vi "Stitch on X axis.vi"(7 "Enum":T1(ring), 8 "error in (no error)":errorcluster, 9 "Right Video":T2, 10 "Initial frame":bool, 11 "Left Video":T2) -> (0 "error out":errorcluster, 3 "Resulting video":T2)   [LabVIEW 2013]
uses:
  <vilib>/vision/Image Controls.llb/IMAQ Image.ctl
  <vilib>/vision/NI_Vision_Development_Module.lvlib
panel:
  # "RE-ENTRANT VI"
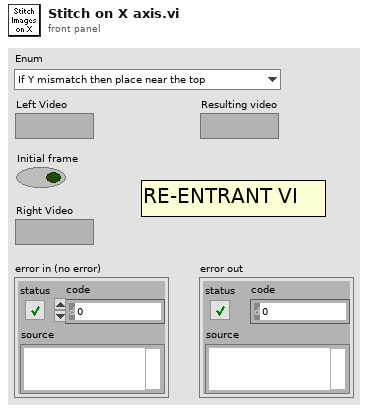
[diagram p1: front panel]
types:
  T1 = enum16{"If Y mismatch then place near the top", "If Y mismatch then place near the bottom"}
  T2 = typedef "IMAQ Image.ctl" = refnum<image>
  T3 = typedef "Image Type" = u32
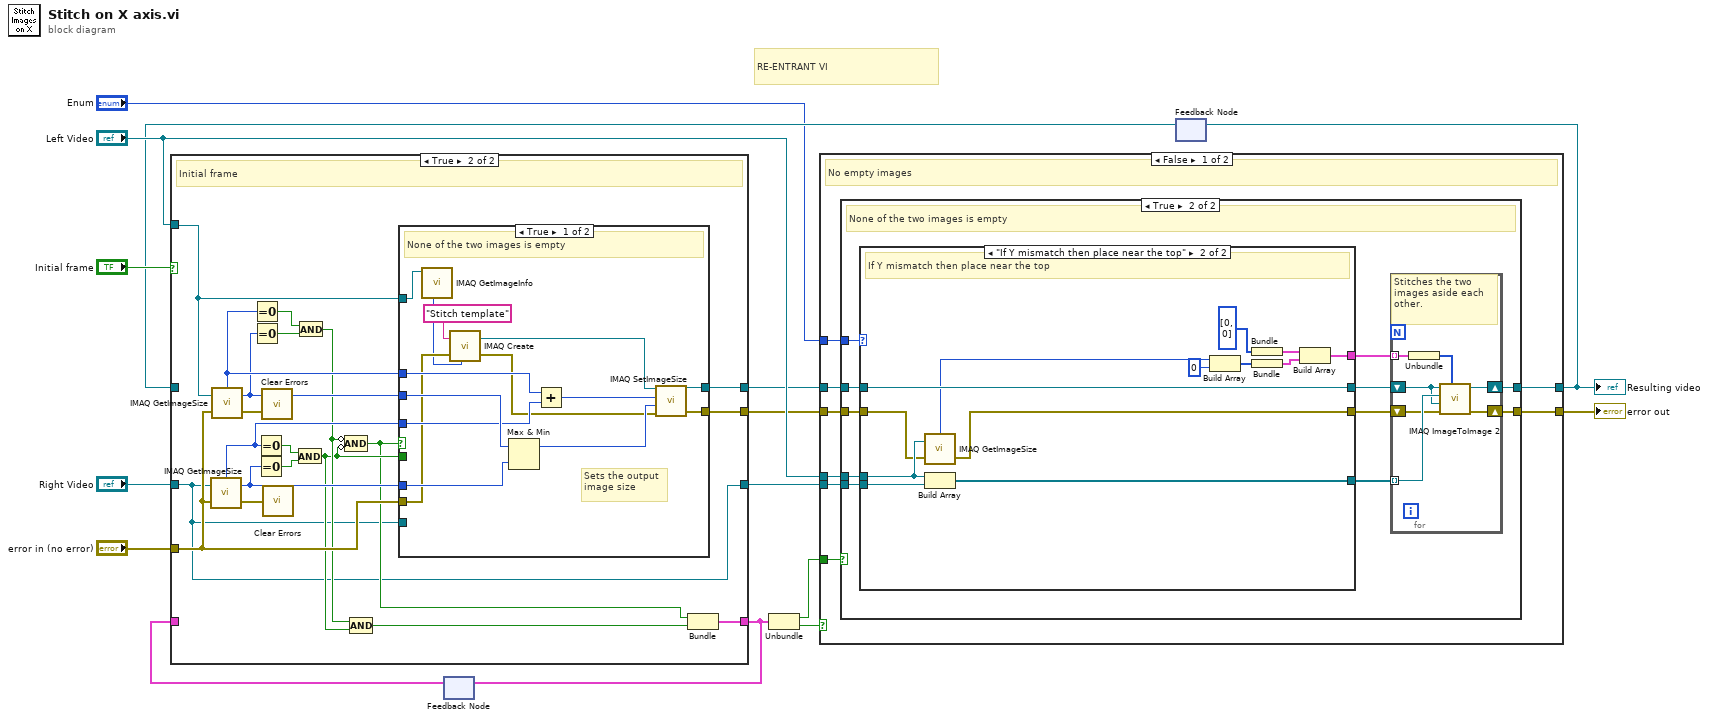
[diagram p0: block diagram]
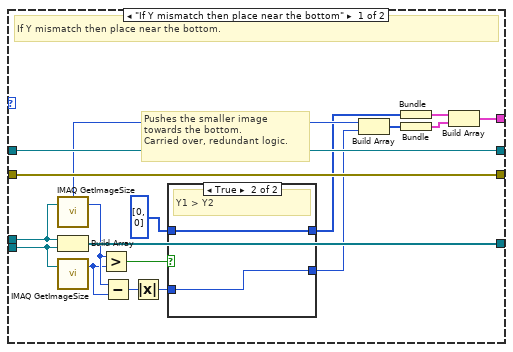
[diagram p3: hidden frame]
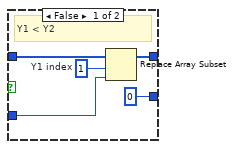
[diagram p4: hidden frame]
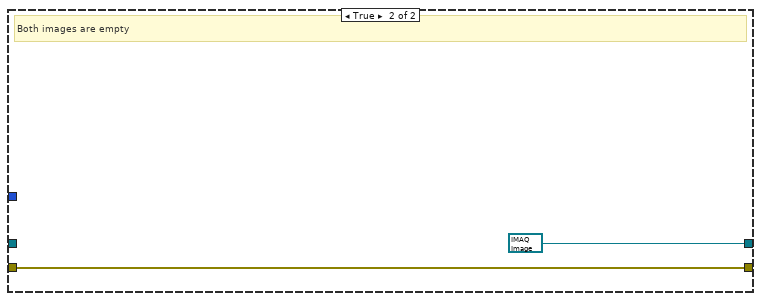
[diagram p5: hidden frame]
diagram:
  # "RE-ENTRANT VI"
  n1 = feedback #1() -> (w8:cluster{bool, bool})  [unwired: 1 in]
  n2 = feedback #2() -> (w7:T2)  [unwired: 1 in]
  n3 = case shown="True" "Initial frame" {
    tunnel: "error in (no error)" -> [w19 w29]
    tunnel: [w19 w38] -> w2
    tunnel: [w18 w39] -> w3
    tunnel: [w17 w20] -> w4
    tunnel: w7 -> [w18 _]
    tunnel: "Right Video" -> [w17 w20]
    tunnel: "Left Video" -> [_ w21]
    tunnel: w8 -> [w16 _]
    tunnel: [w16 w22] -> w9
    frame False {
      # "Default..."
    }
    frame True {
      # "Initial frame"
      n4 = call "IMAQ GetImageSize"("Image"=w20, "error in (no error)"=w29) -> ("Y Resolution"=w31:i32, "X Resolution"=w30:i32, "error out"=w28:errorcluster)  [unwired: 2 in]
      n5 = call "IMAQ GetImageSize"("Image"=w21, "error in (no error)"=w29) -> ("Y Resolution"=w36:i32, "X Resolution"=w37:i32, "error out"=w27:errorcluster)  [unwired: 2 in]
      n6 = Equal To 0?(x=w37) -> (x = 0?=w35:bool)
      n7 = Equal To 0?(x=w36) -> (x = 0?=w34:bool)
      n8 = Equal To 0?(x=w30) -> (x = 0?=w33:bool)
      n9 = Equal To 0?(x=w31) -> (x = 0?=w32:bool)
      n10 = call <vilib>:"Clear Errors.vi"("error in (no error)"=w27) -> ()  [unwired: 6 in, 1 out]
      n11 = call <vilib>:"Clear Errors.vi"("error in (no error)"=w28) -> ()  [unwired: 6 in, 1 out]
      n12 = And(x=w33, y=w32) -> (x .and. y?=w25:bool)
      n13 = And(x=w35, y=w34) -> (x .and. y?=w26:bool)
      n14 = Compound Arithmetic op=AND(invert w26, invert w25) -> (w24:bool)
      n15 = Compound Arithmetic op=AND(w26, w25) -> (w23:bool)
      n16 = case shown="True" w24 {
        tunnel: [w53 w63] -> w39
        tunnel: w29 -> [w43 w62]
        tunnel: [w52 w61] -> w38
        tunnel: w37 -> [w51 w60]
        tunnel: w36 -> [w50 w59]
        tunnel: w31 -> [w49 w58]
        tunnel: w30 -> [w48 w57]
        tunnel: w25 -> [_ w56]
        tunnel: w21 -> [w41 w55]
        tunnel: w20 -> [_ w54]
        frame True {
          # "Sets the output image size"
          # "None of the two images is empty"
          n17 = call "IMAQ GetImageInfo"("Image"=w41) -> ("Image Type"=w40:T3)  [unwired: 3 in, 7 out]
          n18 = call "IMAQ Create"("Image Name"="Stitch template", "Image Type"=w40, "error in (no error)"=w43) -> ("New Image"=w45:T2, "error out"=w44:errorcluster)  [unwired: 1 in, 1 out]
          n19 = Max & Min(x=w50, y=w49) -> (max(x,y)=w46:i32)  [unwired: 1 out]
          n20 = Add(x=w51, y=w48) -> (x+y=w47:i32)
          n21 = call "IMAQ SetImageSize"("error in (no error)"=w44, "Y Resolution"=w46, "X Resolution"=w47, "Image"=w45) -> ("error out"=w52:errorcluster, "Image Out"=w53:T2)  [unwired: 1 out]
        }
        frame False {
          # "One or both images are empty."
          n22 = case shown="True" w56 {
            tunnel: [w65 w66] -> w63
            tunnel: w62 -> [w64 w67]
            tunnel: [w64 w67] -> w61
            tunnel: w60 -> [_ _]
            tunnel: w59 -> [_ _]
            tunnel: w58 -> [_ _]
            tunnel: w57 -> [_ _]
            tunnel: w55 -> [_ w66]
            tunnel: w54 -> [w65 _]
            frame False {
            }
            frame True {
            }
          }
        }
      }
      n23 = Bundle(w24, w23) -> (w22:cluster{bool, bool})  [unwired: 1 in]
    }
  }
  n24 = feedback-in #1(w9) -> ()
  n25 = Unbundle(w9) -> (w10:bool, w11:bool)
  n26 = case shown="False" w11 {
    tunnel: w2 -> [w75 w135]
    tunnel: w3 -> [w74 _]
    tunnel: "Left Video" -> [w73 _]
    tunnel: w4 -> [w72 _]
    tunnel: [w71 w135] -> w5
    tunnel: [w70 T2 refnum ("Selected image")] -> w6
    tunnel: w10 -> [w69 _]
    tunnel: "Enum" -> [w68 _]
    frame False {
      # "No empty images"
      n27 = case shown="True" w69 {
        tunnel: w75 -> [w76 w80]
        tunnel: w74 -> [w77 w82]
        tunnel: w73 -> [_ w85]
        tunnel: w72 -> [_ w84]
        tunnel: [w76 w87] -> w71
        tunnel: [w77 w86] -> w70
        tunnel: w68 -> [_ w78]
        frame False {
          # "One of the images is empty"
        }
        frame True {
          # "None of the two images is empty"
          n28 = case shown="\"If Y mismatch then place near the top\"" w78 {
            tunnel: [w106 w126] -> w88
            tunnel: w85 -> [w105 w125]
            tunnel: w84 -> [w104 w124]
            tunnel: [w103 w123] -> w83
            tunnel: w82 -> [w102 w122]
            tunnel: [w102 w122] -> w81
            tunnel: w80 -> [w101 w121]
            tunnel: [w101 w120] -> w79
            frame "If Y mismatch then place near the bottom" {
              # "Pushes the smaller image towards the bottom.\nCarried over, redundant logic."
              # "If Y mismatch then place near the bottom."
              n29 = call "IMAQ GetImageSize"("Image"=w105) -> ("Y Resolution"=w99:i32, "X Resolution"=w94:i32)  [unwired: 1 in, 3 out]
              n30 = Build Array(w105, w104) -> (w106:T2[])
              n31 = call "IMAQ GetImageSize"("Image"=w104) -> ("Y Resolution"=w98:i32)  [unwired: 1 in, 4 out]
              n32 = Greater?(x=w99, y=w98) -> (0:w100:bool)
              n33 = Subtract(x=w99, y=w98) -> (x-y=w97:i32)
              n34 = Absolute Value(x=w97) -> (abs(x)=w96:i32)
              n35 = case shown="True" w100 {
                tunnel: i32[] [0, 0] -> [w110 w113]
                tunnel: [w109 w113] -> w91
                tunnel: w96 -> [w108 w112]
                tunnel: [0 ("new element/subarray") w112] -> w93
                frame False {
                  w111 = 1  # Y1 index
                  # "Y1 < Y2"
                  n36 = Replace Array Subset(array=w110, new element=w108, index=w111) -> (w109:i32[])
                }
                frame True {
                  # "Y1 > Y2"
                }
              }
              n37 = Build Array(w94, w93) -> (w92:i32[])
              n38 = Bundle(w91) -> (w89:cluster{i32[]})  [unwired: 1 in]
              n39 = Bundle(w92) -> (w90:cluster{i32[]})  [unwired: 1 in]
              n40 = Build Array(w89, w90) -> (w103:cluster{i32[]}[])
            }
            frame "If Y mismatch then place near the top" {
              # "If Y mismatch then place near the top"
              n41 = call "IMAQ GetImageSize"("Image"=w125, "error in (no error)"=w121) -> ("X Resolution"=w119:i32, "error out"=w120:errorcluster)  [unwired: 3 out]
              n42 = Build Array(w125, w124) -> (w126:T2[])
              n43 = Build Array(w119, 0 ("element")) -> (w118:i32[])
              n44 = Bundle(i32[] [0, 0]) -> (w115:cluster{i32[]})  [unwired: 1 in]
              n45 = Bundle(w118) -> (w116:cluster{i32[]})  [unwired: 1 in]
              n46 = Build Array(w115, w116) -> (w123:cluster{i32[]}[])
            }
          }
          n47 = for {
            tunnel: w88 -> [w133] mode=indexing
            shift-right: [w132] -> w86
            shift-left: w81 -> [w131]
            shift-right: [w130] -> w87
            shift-left: w79 -> [w129]
            tunnel: w83 -> [w128] mode=indexing
            # "Stitches the two images aside each other."
            n48 = Unbundle(w128) -> (w127:i32[])
            n49 = call "IMAQ ImageToImage 2"("Offset Left/Top"=w127, "error in (no error)"=w129, "Image Dst"=w131, "Image Src (Small)"=w133, "Image Src (Large)"=w131) -> ("error out"=w130:errorcluster, "Image Dst Out"=w132:T2)  [unwired: 1 in, 4 out]
          }
        }
      }
    }
    frame True {
      # "Both images are empty"
    }
  }
  "Resulting video" <- w6
  "error out" <- w5
  n50 = feedback-in #2(w6) -> ()
